vi "AI config not UI to UI.vi"(11 "AI Config":T2 {"input terminal configuration" items=["default"=-1, "RSE"=10083, "NRSE"=10078, "Differential"=10106, "Pseudodifferential"=12529]; "AI.Coupling" items=["AC"=10045, "DC"=10050, "GND"=10066]}) -> (1 "DAQ Types":T1[](array[typedef]), 2 "input terminal configurations":i32[](array[numeric]), 3 "AI Config (UI)":T6 {"AI.Coupling" items=["AC"=10045, "DC"=10050, "GND"=10066]})   [LabVIEW 2016, in "Instrument.Lockin.lvclass"]
uses:
  Instrument.Lockin.lvclass
  LockinDAQ/Typedefs/AI.config(UI)-array.ctl
  LockinDAQ/Typedefs/AI.config(UI)-cluster.ctl
  LockinDAQ/Typedefs/AI.coupling-enum.ctl
  LockinDAQ/Typedefs/446xAI-enum.ctl
  LockinDAQ/Typedefs/AI.config-array.ctl
  LockinDAQ/Typedefs/AI.config-cluster.ctl
  LockinDAQ/Typedefs/DAQType-enum.ctl
  LockinDAQ/LockinDAQ.lvclass
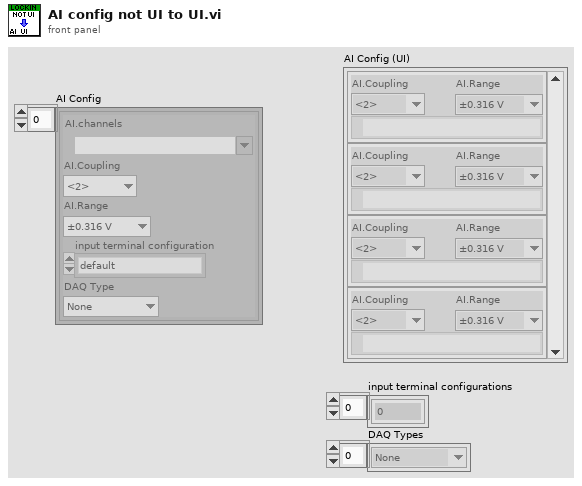
[diagram p1: front panel]
types:
  T1 = typedef "LockinDAQ.lvclass/DAQType-enum.ctl" = enum16{"None", "USB 4431", "PXI 446x"}
  T2 = typedef "LockinDAQ.lvclass/AI.config-array.ctl" = T3[]
  T3 = typedef "LockinDAQ.lvclass/AI.config-cluster.ctl" = cluster{"AI.channels":tag, "AI.Coupling":T4, "AI.Range":T5, "input terminal configuration":i32, "DAQ Type":T1}
  T4 = typedef "LockinDAQ.lvclass/AI.coupling-enum.ctl" = u16
  T5 = typedef "LockinDAQ.lvclass/446xAI-enum.ctl" = enum16{"±0.316 V", "±1.00 V", "±3.16 V", "±10.0 V", "±31.6 V", "±42.4 V"}
  T6 = typedef "LockinDAQ.lvclass/AI.config(UI)-array.ctl" = T7[]
  T7 = typedef "LockinDAQ.lvclass/AI.config(UI)-cluster.ctl" = cluster{"AI.Coupling":T4, "AI.channels":tag, "AI.Range":T5}
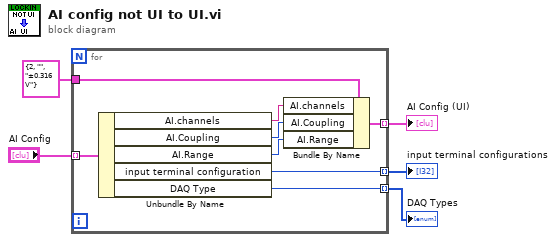
[diagram p0: block diagram]
diagram:
  n1 = for {
    tunnel: T7 {"AI.Coupling"=2, "AI.channels"="", "AI.Range"=enum."±0.316 V"} ("Cluster") -> [w13]
    tunnel: "AI Config" -> [w12] mode=indexing
    tunnel: [w8] -> w5 mode=indexing
    tunnel: [w7] -> w2 mode=indexing
    tunnel: [w6] -> w1 mode=indexing
    n2 = Unbundle By Name(w12) -> ("AI.channels"=w11:tag, "AI.Coupling"=w10:T4, "AI.Range"=w9:T5, "input terminal configuration"=w7:i32, "DAQ Type"=w6:T1)
    n3 = Bundle By Name(cluster=w13, "AI.channels"=w11, "AI.Coupling"=w10, "AI.Range"=w9) -> (w8:T7)
  }
  "AI Config (UI)" <- w5
  "input terminal configurations" <- w2
  "DAQ Types" <- w1
